vi "GateTime.vi"(8 "error in":errorcluster, 9 "Funk_pom":enum32{"F:1", "F:2"}(radio), 10 "stop (F)":bool, 11 "number of samples":i32=100) -> (0 "error out":errorcluster, 2 "stopped":bool, 3 "Czas impulsu":dbl)   [LabVIEW 2021]
panel:
  # "Funkcje pomiarowe"
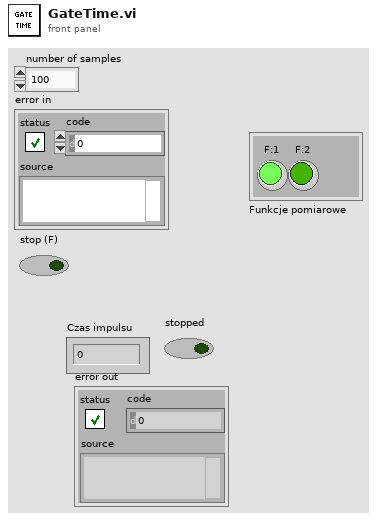
[diagram p1: front panel]
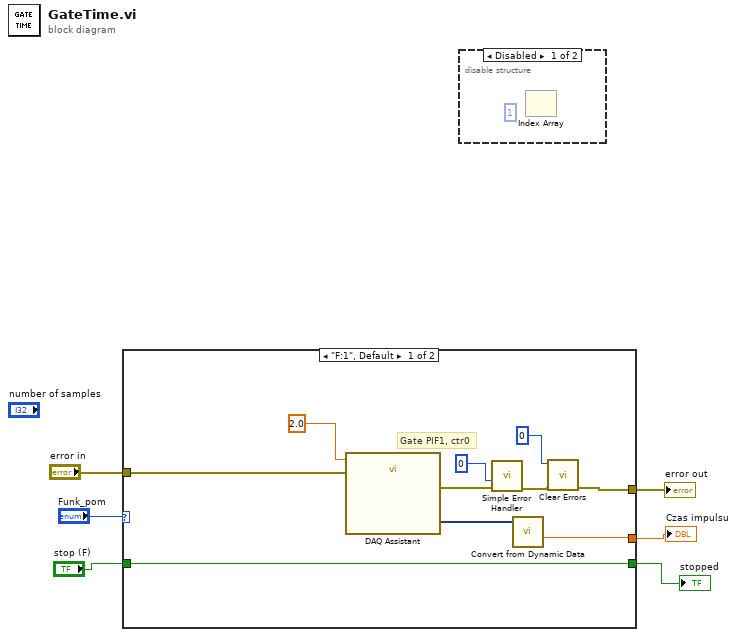
[diagram p0: block diagram]
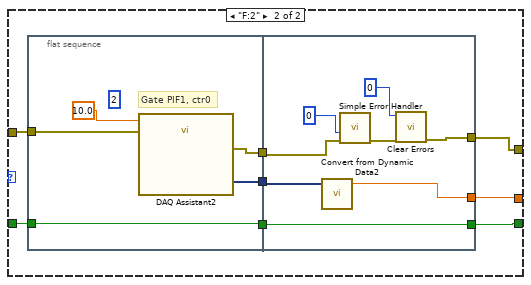
[diagram p2: hidden frame]
diagram:
  n1 = case shown="\"F:1\", Default" "Funk_pom" {
    tunnel: "error in" -> [w14 w24]
    tunnel: "stop (F)" -> [w13 w20]
    tunnel: [w7 w21] -> w3
    tunnel: [w13 w18] -> w2
    tunnel: [w12 w17] -> w1
    frame "F:1", Default {
      # "Gate PIF1, ctr0"
      n2 = call "DAQ Assistant"("timeout (s)"=2.0, "error in"=w14) -> ("data"=w16:dynamicdata, "error out"=w9:errorcluster)  [unwired: 15 in, 1 out]
      n3 = call <vilib>:"Simple Error Handler.vi"("type of dialog (OK msg:1)"=0, "error in (no error)"=w9) -> ("error out"=w8:errorcluster)  [unwired: 3 in, 4 out]
      n4 = call "Convert from Dynamic Data"("Dynamic Data Type"=w16) -> ("Scalar"=w12:dbl)  [unwired: 3 in]
      n5 = call <vilib>:"Clear Errors.vi"("error in (no error)"=w8, "specific error code to clear (0: all)"=0) -> ("error out"=w7:errorcluster)  [unwired: 4 in, 1 out]
    }
    frame "F:2" {
      n6 = flat-sequence {
        tunnel: w24 -> [w27]
        tunnel: [w29] -> w23
        tunnel: [w26] -> w22
        tunnel: w20 -> [w25]
        tunnel: [w25] -> w19
        tunnel: w23 -> [w33]
        tunnel: w22 -> [w34]
        tunnel: [w32] -> w21
        tunnel: w19 -> [w31]
        tunnel: [w31] -> w18
        tunnel: [w30] -> w17
        frame #0 {
          (unwired) 2 ("number of samples")
          # "Gate PIF1, ctr0"
          n7 = call "DAQ Assistant2"("timeout (s)"=10.0, "error in"=w27) -> ("data"=w29:dynamicdata, "error out"=w26:errorcluster)  [unwired: 15 in, 1 out]
        }
        frame #1 {
          n8 = call "Convert from Dynamic Data2"("Dynamic Data Type"=w33) -> ("Scalar"=w30:dbl)  [unwired: 3 in]
          n9 = call <vilib>:"Simple Error Handler.vi"("type of dialog (OK msg:1)"=0, "error in (no error)"=w34) -> ("error out"=w37:errorcluster)  [unwired: 3 in, 4 out]
          n10 = call <vilib>:"Clear Errors.vi"("error in (no error)"=w37, "specific error code to clear (0: all)"=0) -> ("error out"=w32:errorcluster)  [unwired: 4 in, 1 out]
        }
      }
    }
  }
  "error out" <- w3
  "Czas impulsu" <- w1
  "stopped" <- w2
  n11 = disable-structure shown="Disabled" {
    frame Disabled {
      (unwired) 1 ("index")
      n12 = Index Array() -> ()  [unwired: 2 in, 1 out]
    }
    frame Enabled {
    }
  }
